vi "Read Saving.vi"(8 "error in (no error)":errorcluster, 11 "Saving File Message in":refnum<class "Saving File Message.lvclass">) -> (0 "error out":errorcluster, 2 "Saving":bool, 3 "Saving File Message out":refnum<class "Saving File Message.lvclass">)   [LabVIEW 2017, in "File Library.lvlib" / "Saving File Message.lvclass"]
uses:
  Saving File Message.lvclass
  Saving File Message.lvclass/Saving File Message.ctl
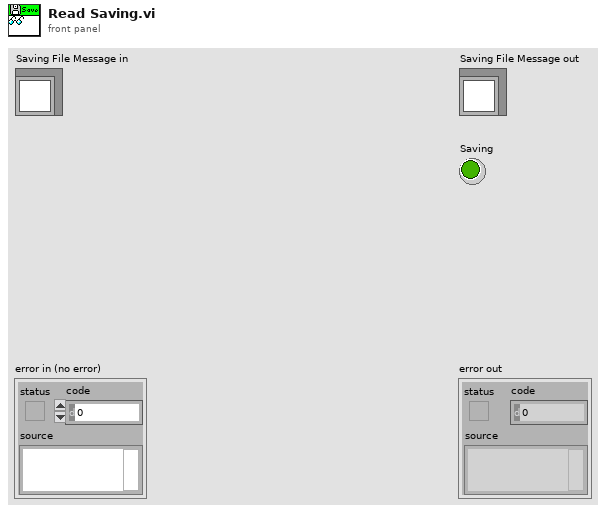
[diagram p1: front panel]
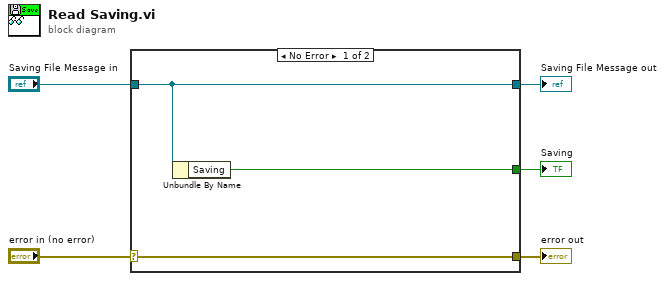
[diagram p0: block diagram]
diagram:
  n1 = case shown="No Error" "error in (no error)" {
    selector: "error in (no error)" -> [w8 w9]
    tunnel: [w8 w9] -> w4
    tunnel: [w7 w10] -> w2
    tunnel: "Saving File Message in" -> [w7 w10]
    tunnel: [w6 _] -> w1
    frame No Error {
      n2 = Unbundle By Name(w7) -> ("Saving"=w6:bool)
    }
    frame Error {
    }
  }
  "error out" <- w4
  "Saving File Message out" <- w2
  "Saving" <- w1
